vi "Dresden Edit Recipe(in).vi"() -> ()   [LabVIEW 2009] (continued)
                    n1472 = property on="R Single RF Step8 Coating Power" class="DigNum (strict)"("DisabledEnum"=w1081) -> ()  [unwired: 2 in, 2 out]
                    n1473 = property on="R Single RF Interval length8" class="DigNum (strict)"("DisabledEnum"=w1081) -> ()  [unwired: 2 in, 2 out]
                  }
                  frame #1 {
                    w1082 = T5."Enabled" ("Disabled")
                    n1474 = property on="R Single RF Step8 Coating Power" class="DigNum (strict)"("DisabledEnum"=w1082) -> ()  [unwired: 2 in, 2 out]
                    n1475 = property on="R Single RF Interval length8" class="DigNum (strict)"("DisabledEnum"=w1082) -> ()  [unwired: 2 in, 2 out]
                  }
                }
              }
            }
            n1476 = Multiply(x=w895, y=w874) -> (x*y=w864:dbl)
            n1477 = Multiply(x=w893, y=w873) -> (x*y=w862:dbl)
            n1478 = Multiply(x=w896, y=w876) -> (x*y=w865:dbl)
            n1479 = Multiply(x=w892, y=w872) -> (x*y=w861:dbl)
            n1480 = case shown="False" w846 {
              frame #0 {
                w1137 = FALSE ("R Single DC Step8 Coating Power Active")
                n1481 = local write "R Single DC Step7 Coating Power Active"(w1137) -> ()
                n1482 = local write "R Single DC Step8 Coating Power Active"(w1137) -> ()
                n1483 = local write "R Single DC Step9 Coating Power Active"(w1137) -> ()
                n1484 = local write "R Single DC Step10 Coating Power Active"(w1137) -> ()
                n1485 = local write "R Single DC Step6 Coating Power Active"(w1137) -> ()
              }
              frame #1 {
                n1486 = local read "R Single DC Step6 Coating Power Active"() -> (w1138:bool)
                n1487 = case shown="False" w1138 {
                  frame #0 {
                    w1139 = 0.0 ("Target Clean Power")
                    w1140 = T5."Disabled and Grayed Out" ("Disabled")
                    n1488 = local write "R Single DC Step6 Coating Power"(w1139) -> ()
                    n1489 = local write "R Single DC Interval length6"(w1139) -> ()
                    n1490 = property on="R Single DC Step6 Coating Power" class="DigNum (strict)"("DisabledEnum"=w1140) -> ()  [unwired: 2 in, 2 out]
                    n1491 = property on="R Single DC Interval length6" class="DigNum (strict)"("DisabledEnum"=w1140) -> ()  [unwired: 2 in, 2 out]
                  }
                  frame #1 {
                    w1141 = T5."Enabled" ("Disabled")
                    n1492 = property on="R Single DC Step6 Coating Power" class="DigNum (strict)"("DisabledEnum"=w1141) -> ()  [unwired: 2 in, 2 out]
                    n1493 = property on="R Single DC Interval length6" class="DigNum (strict)"("DisabledEnum"=w1141) -> ()  [unwired: 2 in, 2 out]
                  }
                }
              }
            }
            n1494 = Multiply(x=w891, y=w871) -> (x*y=w860:dbl)
            n1495 = Multiply(x=w894, y=w875) -> (x*y=w863:dbl)
            n1496 = case shown="False" w845 {
              frame #0 {
                w1132 = FALSE ("R Single DC Step8 Coating Power Active")
                n1497 = local write "R Single DC Step10 Coating Power Active"(w1132) -> ()
                n1498 = local write "R Single DC Step9 Coating Power Active"(w1132) -> ()
                n1499 = local write "R Single DC Step8 Coating Power Active"(w1132) -> ()
                n1500 = local write "R Single DC Step7 Coating Power Active"(w1132) -> ()
              }
              frame #1 {
                n1501 = local read "R Single DC Step7 Coating Power Active"() -> (w1133:bool)
                n1502 = case shown="False" w1133 {
                  frame #0 {
                    w1134 = 0.0 ("Target Clean Power")
                    w1135 = T5."Disabled and Grayed Out" ("Disabled")
                    n1503 = local write "R Single DC Step7 Coating Power"(w1134) -> ()
                    n1504 = local write "R Single DC Interval length7"(w1134) -> ()
                    n1505 = property on="R Single DC Step7 Coating Power" class="DigNum (strict)"("DisabledEnum"=w1135) -> ()  [unwired: 2 in, 2 out]
                    n1506 = property on="R Single DC Interval length7" class="DigNum (strict)"("DisabledEnum"=w1135) -> ()  [unwired: 2 in, 2 out]
                  }
                  frame #1 {
                    w1136 = T5."Enabled" ("Disabled")
                    n1507 = property on="R Single DC Step7 Coating Power" class="DigNum (strict)"("DisabledEnum"=w1136) -> ()  [unwired: 2 in, 2 out]
                    n1508 = property on="R Single DC Interval length7" class="DigNum (strict)"("DisabledEnum"=w1136) -> ()  [unwired: 2 in, 2 out]
                  }
                }
              }
            }
            n1509 = Compound Arithmetic op=ADD(w869, w868, w867, w866, w865, w864, w863, w862, w861, w860) -> (→"Calculated_total_length_cmb":dbl)
            n1510 = case shown="False" w844 {
              frame #0 {
                w1127 = FALSE ("R Single DC Step8 Coating Power Active")
                n1511 = local write "R Single DC Step10 Coating Power Active"(w1127) -> ()
                n1512 = local write "R Single DC Step9 Coating Power Active"(w1127) -> ()
                n1513 = local write "R Single DC Step8 Coating Power Active"(w1127) -> ()
              }
              frame #1 {
                n1514 = local read "R Single DC Step8 Coating Power Active"() -> (w1128:bool)
                n1515 = case shown="False" w1128 {
                  frame #0 {
                    w1129 = 0.0 ("R Single DC Step8 Coating Power")
                    w1130 = T5."Disabled and Grayed Out" ("Disabled")
                    n1516 = local write "R Single DC Step8 Coating Power"(w1129) -> ()
                    n1517 = local write "R Single DC Interval length8"(w1129) -> ()
                    n1518 = property on="R Single DC Step8 Coating Power" class="DigNum (strict)"("DisabledEnum"=w1130) -> ()  [unwired: 2 in, 2 out]
                    n1519 = property on="R Single DC Interval length8" class="DigNum (strict)"("DisabledEnum"=w1130) -> ()  [unwired: 2 in, 2 out]
                  }
                  frame #1 {
                    w1131 = T5."Enabled" ("Disabled")
                    n1520 = property on="R Single DC Step8 Coating Power" class="DigNum (strict)"("DisabledEnum"=w1131) -> ()  [unwired: 2 in, 2 out]
                    n1521 = property on="R Single DC Interval length8" class="DigNum (strict)"("DisabledEnum"=w1131) -> ()  [unwired: 2 in, 2 out]
                  }
                }
              }
            }
            n1522 = case shown="True" "Power_list_open_multi" {
              frame #0 {
                n1523 = property on="Multilayer_power_tab" class="TabCtl (strict)"("Visible"=FALSE) -> ()  [unwired: 2 in, 2 out]
              }
              frame #1 {
                n1524 = property on="Multilayer_power_tab" class="TabCtl (strict)"("Visible"=TRUE) -> ()  [unwired: 2 in, 2 out]
              }
            }
            n1525 = stacked-sequence {
              frame #0 {
                # "Thickness Monitor Parameters Set"
                n1526 = local read "R_Single DC_Material ok"() -> (w1960:bool)
                n1527 = local read "R_Single RF Material ok"() -> (w1959:bool)
                n1528 = local read "R_Cmb Ch2_Material ok"() -> (w1958:bool)
                n1529 = local read "R Cmb Ch3 Material ok"() -> (w1957:bool)
                n1530 = Build Array(FALSE, w1960, w1959, w1958, w1957) -> (w1978:bool[])
                n1531 = Boolean Array To Number(Boolean array=w1978) -> (number=w1977:u32)
                n1532 = Mantissa & Exponent(0:w1977) -> (2:w1975:dbl)  [unwired: 1 out]
                n1533 = case shown="0, Default" w1975 {
                  tunnel: ["" ("Evs_1_mat") w2030 w2032 w2034 w2036] -> w1968
                  frame #0 {
                  }
                  frame #1 {
                    n1534 = local read "R Single DC Target material"() -> (w2030:string)
                    n1535 = local write "R_Single DC_Material ok"(FALSE ("R_Single DC_Material ok")) -> ()
                  }
                  frame #2 {
                    n1536 = local read "R Single RF Target material"() -> (w2032:string)
                    n1537 = local write "R_Single RF Material ok"(FALSE ("R_Single RF Material ok")) -> ()
                  }
                  frame #3 {
                    n1538 = local read "R Cmb Ch2 Target material"() -> (w2034:string)
                    n1539 = local write "R_Cmb Ch2_Material ok"(FALSE ("R_Cmb Ch2_Material ok")) -> ()
                  }
                  frame #4 {
                    n1540 = local read "R Cmb Ch3 Target material"() -> (w2036:string)
                    n1541 = local write "R Cmb Ch3 Material ok"(FALSE ("R Cmb Ch3 Material ok")) -> ()
                  }
                }
                n1542 = local read "R_Single DC_Material ok"() -> (w1956:bool)
                n1543 = local read "R_Single RF Material ok"() -> (w1955:bool)
                n1544 = local read "R_Cmb Ch2_Material ok"() -> (w1954:bool)
                n1545 = local read "R Cmb Ch3 Material ok"() -> (w1953:bool)
                n1546 = Read from Text File(file (use dialog)=path "D:/VK-1701 System Files/Material/Material Properties.txt") -> (text=w1973:string)  [unwired: 3 in, 3 out]
                n1547 = Match Pattern(string=w1973, regular expression=w1968) -> (after substring=w1974:string)  [unwired: 1 in, 3 out]
                n1548 = String Length(string=w1968) -> (length=w1969:i32)
                n1549 = Build Array(FALSE, w1956, w1955, w1954, w1953) -> (w1965:bool[])
                n1550 = Match Pattern(string=w1974, regular expression="=") -> (after substring=w1972:string)  [unwired: 1 in, 3 out]
                n1551 = Boolean Array To Number(Boolean array=w1965) -> (number=w1966:u32)
                n1552 = Not Equal To 0?(x=w1969) -> (x != 0?=w1963:bool)
                n1553 = Match Pattern(string=w1972, regular expression="***") -> (before substring=w1962:string)  [unwired: 1 in, 3 out]
                n1554 = Mantissa & Exponent(0:w1966) -> (2:w1961:dbl)  [unwired: 1 out]
                n1555 = case shown="True" w1963 {
                  tunnel: w1962 -> [_ w1979]
                  tunnel: w1961 -> [_ w1980]
                  frame #0 {
                  }
                  frame #1 {
                    n1556 = case shown="3" w1980 {
                      tunnel: w1979 -> [_ w1981 w1993 w2005 w2017]
                      frame #0 {
                      }
                      frame #1 {
                        n1557 = String Subset(string=w1981, offset (0)=4, length (rest)=5 ("length (rest)")) -> (substring=w1992:string)
                        n1558 = String Subset(string=w1981, offset (0)=0, length (rest)=4 ("length (rest)")) -> (substring=w1990:string)
                        n1559 = Scan Value(string=w1992, format string="%.3f") -> (value=w1982:dbl)  [unwired: 1 in, 1 out]
                        n1560 = Scan Value(string=w1990, format string="%.2f") -> (value=w1984:dbl)  [unwired: 1 in, 1 out]
                        n1561 = local write "R Z_factor"(w1982) -> ()
                        n1562 = local write "R Material_density"(w1984) -> ()
                        n1563 = local write "R Toooling_factor"(0.0 ("R Toooling_factor")) -> ()
                      }
                      frame #2 {
                        n1564 = String Subset(string=w1993, offset (0)=4, length (rest)=5 ("length (rest)")) -> (substring=w2004:string)
                        n1565 = String Subset(string=w1993, offset (0)=0, length (rest)=4 ("length (rest)")) -> (substring=w2002:string)
                        n1566 = Scan Value(string=w2004, format string="%.3f") -> (value=w1994:dbl)  [unwired: 1 in, 1 out]
                        n1567 = Scan Value(string=w2002, format string="%.2f") -> (value=w1996:dbl)  [unwired: 1 in, 1 out]
                        n1568 = local write "R Z_factor"(w1994) -> ()
                        n1569 = local write "R Material_density"(w1996) -> ()
                        n1570 = local write "R Toooling_factor"(0.0 ("R Toooling_factor")) -> ()
                      }
                      frame #3 {
                        n1571 = String Subset(string=w2005, offset (0)=4, length (rest)=5 ("length (rest)")) -> (substring=w2016:string)
                        n1572 = String Subset(string=w2005, offset (0)=0, length (rest)=4 ("length (rest)")) -> (substring=w2014:string)
                        n1573 = Scan Value(string=w2016, format string="%.3f") -> (value=w2006:dbl)  [unwired: 1 in, 1 out]
                        n1574 = Scan Value(string=w2014, format string="%.2f") -> (value=w2008:dbl)  [unwired: 1 in, 1 out]
                        n1575 = local write "R Z_factor"(w2006) -> ()
                        n1576 = local write "R Material_density"(w2008) -> ()
                        n1577 = local write "R Toooling_factor"(0.0 ("R Toooling_factor")) -> ()
                      }
                      frame #4 {
                        n1578 = String Subset(string=w2017, offset (0)=4, length (rest)=5 ("length (rest)")) -> (substring=w2028:string)
                        n1579 = String Subset(string=w2017, offset (0)=0, length (rest)=4 ("length (rest)")) -> (substring=w2026:string)
                        n1580 = Scan Value(string=w2028, format string="%.3f") -> (value=w2018:dbl)  [unwired: 1 in, 1 out]
                        n1581 = Scan Value(string=w2026, format string="%.2f") -> (value=w2020:dbl)  [unwired: 1 in, 1 out]
                        n1582 = local write "R Z_factor"(w2018) -> ()
                        n1583 = local write "R Material_density"(w2020) -> ()
                        n1584 = local write "R Toooling_factor"(0.0 ("R Toooling_factor")) -> ()
                      }
                    }
                  }
                }
              }
            }
            n1585 = local read "R Cmb Step2 Coating Power Active"() -> (w831:bool)
            n1586 = local read "R Cmb Step1 Coating Power Active"() -> (w832:bool)
            n1587 = local read "R Cmb Step4 Coating Power Active"() -> (w829:bool)
            n1588 = local read "Recipe_selection tab"() -> (w986:T1)
            n1589 = local read "R Cmb Step3 Coating Power Active"() -> (w830:bool)
            n1590 = case shown="100" "R_Single DC_Mat_sel" {
              frame #0 {
              }
              frame #1 {
                n1591 = local write "R Single DC Target material"("Ag" ("R DC Target material")) -> ()
              }
              frame #2 {
                n1592 = local write "R Single DC Target material"("AgBr" ("R DC Target material")) -> ()
              }
              frame #3 {
                n1593 = local write "R Single DC Target material"("AgCl" ("R DC Target material")) -> ()
              }
              frame #4 {
                n1594 = local write "R Single DC Target material"("Al" ("R DC Target material")) -> ()
              }
              frame #5 {
                n1595 = local write "R Single DC Target material"("Al2O3" ("R DC Target material")) -> ()
              }
              frame #6 {
                n1596 = local write "R Single DC Target material"("As" ("R DC Target material")) -> ()
              }
              frame #7 {
                n1597 = local write "R Single DC Target material"("Au" ("R DC Target material")) -> ()
              }
              frame #8 {
                n1598 = local write "R Single DC Target material"("B" ("R DC Target material")) -> ()
              }
              frame #9 {
                n1599 = local write "R Single DC Target material"("Ba" ("R DC Target material")) -> ()
              }
              frame #10 {
                n1600 = local write "R Single DC Target material"("Be" ("R DC Target material")) -> ()
              }
              frame #11 {
                n1601 = local write "R Single DC Target material"("Bi" ("R DC Target material")) -> ()
              }
              frame #12 {
                n1602 = local write "R Single DC Target material"("Bi2O3" ("R DC Target material")) -> ()
              }
              frame #13 {
                n1603 = local write "R Single DC Target material"("C (Diamond)" ("R DC Target material")) -> ()
              }
              frame #14 {
                n1604 = local write "R Single DC Target material"("C (Graphite)" ("R DC Target material")) -> ()
              }
              frame #15 {
                n1605 = local write "R Single DC Target material"("Ca" ("R DC Target material")) -> ()
              }
              frame #16 {
                n1606 = local write "R Single DC Target material"("CaF" ("R DC Target material")) -> ()
              }
              frame #17 {
                n1607 = local write "R Single DC Target material"("Cd" ("R DC Target material")) -> ()
              }
              frame #18 {
                n1608 = local write "R Single DC Target material"("CdS" ("R DC Target material")) -> ()
              }
              frame #19 {
                n1609 = local write "R Single DC Target material"("CdSe" ("R DC Target material")) -> ()
              }
              frame #20 {
                n1610 = local write "R Single DC Target material"("CdTe" ("R DC Target material")) -> ()
              }
              frame #21 {
                n1611 = local write "R Single DC Target material"("CeF3" ("R DC Target material")) -> ()
              }
              frame #22 {
                n1612 = local write "R Single DC Target material"("CeO" ("R DC Target material")) -> ()
              }
              frame #23 {
                n1613 = local write "R Single DC Target material"("Cr" ("R DC Target material")) -> ()
              }
              frame #24 {
                n1614 = local write "R Single DC Target material"("Cr2O3" ("R DC Target material")) -> ()
              }
              frame #25 {
                n1615 = local write "R Single DC Target material"("Co" ("R DC Target material")) -> ()
              }
              frame #26 {
                n1616 = local write "R Single DC Target material"("Cu" ("R DC Target material")) -> ()
              }
              frame #27 {
                n1617 = local write "R Single DC Target material"("Cu2S (A)" ("R DC Target material")) -> ()
              }
              frame #28 {
                n1618 = local write "R Single DC Target material"("Cu2S (B)" ("R DC Target material")) -> ()
              }
              frame #29 {
                n1619 = local write "R Single DC Target material"("CuS" ("R DC Target material")) -> ()
              }
              frame #30 {
                n1620 = local write "R Single DC Target material"("Dy" ("R DC Target material")) -> ()
              }
              frame #31 {
                n1621 = local write "R Single DC Target material"("Er" ("R DC Target material")) -> ()
              }
              frame #32 {
                n1622 = local write "R Single DC Target material"("Fe" ("R DC Target material")) -> ()
              }
              frame #33 {
                n1623 = local write "R Single DC Target material"("Ga" ("R DC Target material")) -> ()
              }
              frame #34 {
                n1624 = local write "R Single DC Target material"("GaAs" ("R DC Target material")) -> ()
              }
              frame #35 {
                n1625 = local write "R Single DC Target material"("Gd" ("R DC Target material")) -> ()
              }
              frame #36 {
                n1626 = local write "R Single DC Target material"("Ge" ("R DC Target material")) -> ()
              }
              frame #37 {
                n1627 = local write "R Single DC Target material"("Hf" ("R DC Target material")) -> ()
              }
              frame #38 {
                n1628 = local write "R Single DC Target material"("HfO2" ("R DC Target material")) -> ()
              }
              frame #39 {
                n1629 = local write "R Single DC Target material"("Hg" ("R DC Target material")) -> ()
              }
              frame #40 {
                n1630 = local write "R Single DC Target material"("Ho" ("R DC Target material")) -> ()
              }
              frame #41 {
                n1631 = local write "R Single DC Target material"("In" ("R DC Target material")) -> ()
              }
              frame #42 {
                n1632 = local write "R Single DC Target material"("InSb" ("R DC Target material")) -> ()
              }
              frame #43 {
                n1633 = local write "R Single DC Target material"("In2O3" ("R DC Target material")) -> ()
              }
              frame #44 {
                n1634 = local write "R Single DC Target material"("Ir" ("R DC Target material")) -> ()
              }
              frame #45 {
                n1635 = local write "R Single DC Target material"("KCl" ("R DC Target material")) -> ()
              }
              frame #46 {
                n1636 = local write "R Single DC Target material"("La" ("R DC Target material")) -> ()
              }
              frame #47 {
                n1637 = local write "R Single DC Target material"("LaF3" ("R DC Target material")) -> ()
              }
              frame #48 {
                n1638 = local write "R Single DC Target material"("LaO3" ("R DC Target material")) -> ()
              }
              frame #49 {
                n1639 = local write "R Single DC Target material"("Li" ("R DC Target material")) -> ()
              }
              frame #50 {
                n1640 = local write "R Single DC Target material"("LiF" ("R DC Target material")) -> ()
              }
              frame #51 {
                n1641 = local write "R Single DC Target material"("Mg" ("R DC Target material")) -> ()
              }
              frame #52 {
                n1642 = local write "R Single DC Target material"("MgF2" ("R DC Target material")) -> ()
              }
              frame #53 {
                n1643 = local write "R Single DC Target material"("MgO" ("R DC Target material")) -> ()
              }
              frame #54 {
                n1644 = local write "R Single DC Target material"("Mn" ("R DC Target material")) -> ()
              }
              frame #55 {
                n1645 = local write "R Single DC Target material"("MnS" ("R DC Target material")) -> ()
              }
              frame #56 {
                n1646 = local write "R Single DC Target material"("Mo" ("R DC Target material")) -> ()
              }
              frame #57 {
                n1647 = local write "R Single DC Target material"("Na" ("R DC Target material")) -> ()
              }
              frame #58 {
                n1648 = local write "R Single DC Target material"("NaCl" ("R DC Target material")) -> ()
              }
              frame #59 {
                n1649 = local write "R Single DC Target material"("NdF3" ("R DC Target material")) -> ()
              }
              frame #60 {
                n1650 = local write "R Single DC Target material"("Nd2O3" ("R DC Target material")) -> ()
              }
              frame #61 {
                n1651 = local write "R Single DC Target material"("Ni" ("R DC Target material")) -> ()
              }
              frame #62 {
                n1652 = local write "R Single DC Target material"("Nb" ("R DC Target material")) -> ()
              }
              frame #63 {
                n1653 = local write "R Single DC Target material"("Nb2O5" ("R DC Target material")) -> ()
              }
              frame #64 {
                n1654 = local write "R Single DC Target material"("Pb" ("R DC Target material")) -> ()
              }
              frame #65 {
                n1655 = local write "R Single DC Target material"("PbS" ("R DC Target material")) -> ()
              }
              frame #66 {
                n1656 = local write "R Single DC Target material"("Pd" ("R DC Target material")) -> ()
              }
              frame #67 {
                n1657 = local write "R Single DC Target material"("Pt" ("R DC Target material")) -> ()
              }
              frame #68 {
                n1658 = local write "R Single DC Target material"("Re" ("R DC Target material")) -> ()
              }
              frame #69 {
                n1659 = local write "R Single DC Target material"("Rh" ("R DC Target material")) -> ()
              }
              frame #70 {
                n1660 = local write "R Single DC Target material"("Rb" ("R DC Target material")) -> ()
              }
              frame #71 {
                n1661 = local write "R Single DC Target material"("S" ("R DC Target material")) -> ()
              }
              frame #72 {
                n1662 = local write "R Single DC Target material"("Sb" ("R DC Target material")) -> ()
              }
              frame #73 {
                n1663 = local write "R Single DC Target material"("Sc" ("R DC Target material")) -> ()
              }
              frame #74 {
                n1664 = local write "R Single DC Target material"("Se" ("R DC Target material")) -> ()
              }
              frame #75 {
                n1665 = local write "R Single DC Target material"("Si" ("R DC Target material")) -> ()
              }
              frame #76 {
                n1666 = local write "R Single DC Target material"("SiO" ("R DC Target material")) -> ()
              }
              frame #77 {
                n1667 = local write "R Single DC Target material"("SiO2" ("R DC Target material")) -> ()
              }
              frame #78 {
                n1668 = local write "R Single DC Target material"("Sm" ("R DC Target material")) -> ()
              }
              frame #79 {
                n1669 = local write "R Single DC Target material"("Sn" ("R DC Target material")) -> ()
              }
              frame #80 {
                n1670 = local write "R Single DC Target material"("Ta" ("R DC Target material")) -> ()
              }
              frame #81 {
                n1671 = local write "R Single DC Target material"("Ta2O5" ("R DC Target material")) -> ()
              }
              frame #82 {
                n1672 = local write "R Single DC Target material"("Te" ("R DC Target material")) -> ()
              }
              frame #83 {
                n1673 = local write "R Single DC Target material"("Tb" ("R DC Target material")) -> ()
              }
              frame #84 {
                n1674 = local write "R Single DC Target material"("ThF4" ("R DC Target material")) -> ()
              }
              frame #85 {
                n1675 = local write "R Single DC Target material"("Ti" ("R DC Target material")) -> ()
              }
              frame #86 {
                n1676 = local write "R Single DC Target material"("TiO2" ("R DC Target material")) -> ()
              }
              frame #87 {
                n1677 = local write "R Single DC Target material"("TiO" ("R DC Target material")) -> ()
              }
              frame #88 {
                n1678 = local write "R Single DC Target material"("Tl" ("R DC Target material")) -> ()
              }
              frame #89 {
                n1679 = local write "R Single DC Target material"("U" ("R DC Target material")) -> ()
              }
              frame #90 {
                n1680 = local write "R Single DC Target material"("V" ("R DC Target material")) -> ()
              }
              frame #91 {
                n1681 = local write "R Single DC Target material"("W" ("R DC Target material")) -> ()
              }
              frame #92 {
                n1682 = local write "R Single DC Target material"("WC" ("R DC Target material")) -> ()
              }
              frame #93 {
                n1683 = local write "R Single DC Target material"("Y" ("R DC Target material")) -> ()
              }
              frame #94 {
                n1684 = local write "R Single DC Target material"("Y2O3" ("R DC Target material")) -> ()
              }
              frame #95 {
                n1685 = local write "R Single DC Target material"("Yb" ("R DC Target material")) -> ()
              }
              frame #96 {
                n1686 = local write "R Single DC Target material"("Zn" ("R DC Target material")) -> ()
              }
              frame #97 {
                n1687 = local write "R Single DC Target material"("ZnO" ("R DC Target material")) -> ()
              }
              frame #98 {
                n1688 = local write "R Single DC Target material"("ZnSe" ("R DC Target material")) -> ()
              }
              frame #99 {
                n1689 = local write "R Single DC Target material"("ZnS" ("R DC Target material")) -> ()
              }
              frame #100 {
                n1690 = local write "R Single DC Target material"("Zr" ("R DC Target material")) -> ()
              }
              frame #101 {
                n1691 = local write "R Single DC Target material"("ZrO2" ("R DC Target material")) -> ()
              }
              frame #102 {
                n1692 = local write "R Single DC Target material"("Si3N4" ("R DC Target material")) -> ()
              }
              frame #103 {
                n1693 = local write "R Single DC Target material"("ITO" ("R DC Target material")) -> ()
              }
              frame #104 {
                n1694 = local write "R Single DC Target material"("PbI2" ("R DC Target material")) -> ()
              }
            }
            n1695 = case shown="1" "R_Cmb Ch2_Mat_sel" {
              frame #0 {
              }
              frame #1 {
                n1696 = local write "R Cmb Ch2 Target material"("Ag" ("R DC Target material")) -> ()
              }
              frame #2 {
                n1697 = local write "R Cmb Ch2 Target material"("AgBr" ("R DC Target material")) -> ()
              }
              frame #3 {
                n1698 = local write "R Cmb Ch2 Target material"("AgCl" ("R DC Target material")) -> ()
              }
              frame #4 {
                n1699 = local write "R Cmb Ch2 Target material"("Al" ("R DC Target material")) -> ()
              }
              frame #5 {
                n1700 = local write "R Cmb Ch2 Target material"("Al2O3" ("R DC Target material")) -> ()
              }
              frame #6 {
                n1701 = local write "R Cmb Ch2 Target material"("As" ("R DC Target material")) -> ()
              }
              frame #7 {
                n1702 = local write "R Cmb Ch2 Target material"("Au" ("R DC Target material")) -> ()
              }
              frame #8 {
                n1703 = local write "R Single DC Target material"("B" ("R DC Target material")) -> ()
              }
              frame #9 {
                n1704 = local write "R Cmb Ch2 Target material"("Ba" ("R DC Target material")) -> ()
              }
              frame #10 {
                n1705 = local write "R Cmb Ch2 Target material"("Be" ("R DC Target material")) -> ()
              }
              frame #11 {
                n1706 = local write "R Cmb Ch2 Target material"("Bi" ("R DC Target material")) -> ()
              }
              frame #12 {
                n1707 = local write "R Cmb Ch2 Target material"("Bi2O3" ("R DC Target material")) -> ()
              }
              frame #13 {
                n1708 = local write "R Cmb Ch2 Target material"("C (Diamond)" ("R DC Target material")) -> ()
              }
              frame #14 {
                n1709 = local write "R Cmb Ch2 Target material"("C (Graphite)" ("R DC Target material")) -> ()
              }
              frame #15 {
                n1710 = local write "R Cmb Ch2 Target material"("Ca" ("R DC Target material")) -> ()
              }
              frame #16 {
                n1711 = local write "R Cmb Ch2 Target material"("CaF" ("R DC Target material")) -> ()
              }
              frame #17 {
                n1712 = local write "R Cmb Ch2 Target material"("Cd" ("R DC Target material")) -> ()
              }
              frame #18 {
                n1713 = local write "R Cmb Ch2 Target material"("CdS" ("R DC Target material")) -> ()
              }
              frame #19 {
                n1714 = local write "R Cmb Ch2 Target material"("CdSe" ("R DC Target material")) -> ()
              }
              frame #20 {
                n1715 = local write "R Cmb Ch2 Target material"("CdTe" ("R DC Target material")) -> ()
              }
              frame #21 {
                n1716 = local write "R Cmb Ch2 Target material"("CeF3" ("R DC Target material")) -> ()
              }
              frame #22 {
                n1717 = local write "R Cmb Ch2 Target material"("CeO" ("R DC Target material")) -> ()
              }
              frame #23 {
                n1718 = local write "R Cmb Ch2 Target material"("Cr" ("R DC Target material")) -> ()
              }
              frame #24 {
                n1719 = local write "R Cmb Ch2 Target material"("Cr2O3" ("R DC Target material")) -> ()
